vi "RPT_Report Calibrate.vi"(8 "template":path=path "C:/AllenProjects/PWC-OLS/$Calibrtation/CAL_Level_RnR_241105.xlsx", 9 "Info":cluster{"Name":string, "Date":string}[](array[cluster])=[{"Name"="Joe", "Date"="Today"}], 10 "LinEq":T1(array[cluster]), 11 "Calibration":cluster{"SP":dbl, "Laser":dbl, "Measure":dbl}[](array[cluster])=[{"SP"=2.0, "Laser"=2.0014999999999996, "Measure"=2.0}, {"SP"=3.5, "Laser"=3.5015, "Measure"=3.5}, {"SP"=5.0, "Laser"=5.001499999999945, "Measure"=5.0}, {"SP"=6.5, "Laser"=6.50149999999989, "Measure"=6.5}, {"SP"=8.0, "Laser"=8.001499999999835, "Measure"=8.0}]) -> ()   [LabVIEW 2024]
uses:
  <vilib>/Utility/NIReport.llb/Report Type.ctl
  <vilib>/addons/_office/excel.llb/Excel Easy Table (str).vi
  <vilib>/Utility/NIReport.llb/NI_report.lvclass
  <vilib>/Utility/NIReport.llb/NI_ReportGenerationCore.lvlib
  <vilib>/Utility/NIReport.llb/Excel/NI_Excel.lvclass
  <vilib>/addons/_office/NI_ReportGenerationToolkit.lvlib
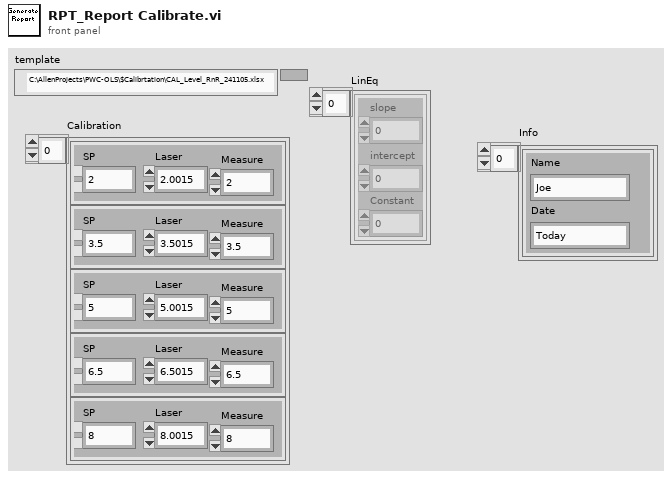
[diagram p1: front panel]
types:
  T1 = cluster{"slope":dbl, "intercept":dbl, "Constant":dbl}[]
  T2 = typedef "NI_ReportGenerationCore.lvlib/Report Type.ctl" = enum16{"HTML", "Word", "Excel"}
  T3 = cluster{"position (excel)":cluster{"row":i32, "column":i32}, "name (excel)":string, "bookmark (word)":string}
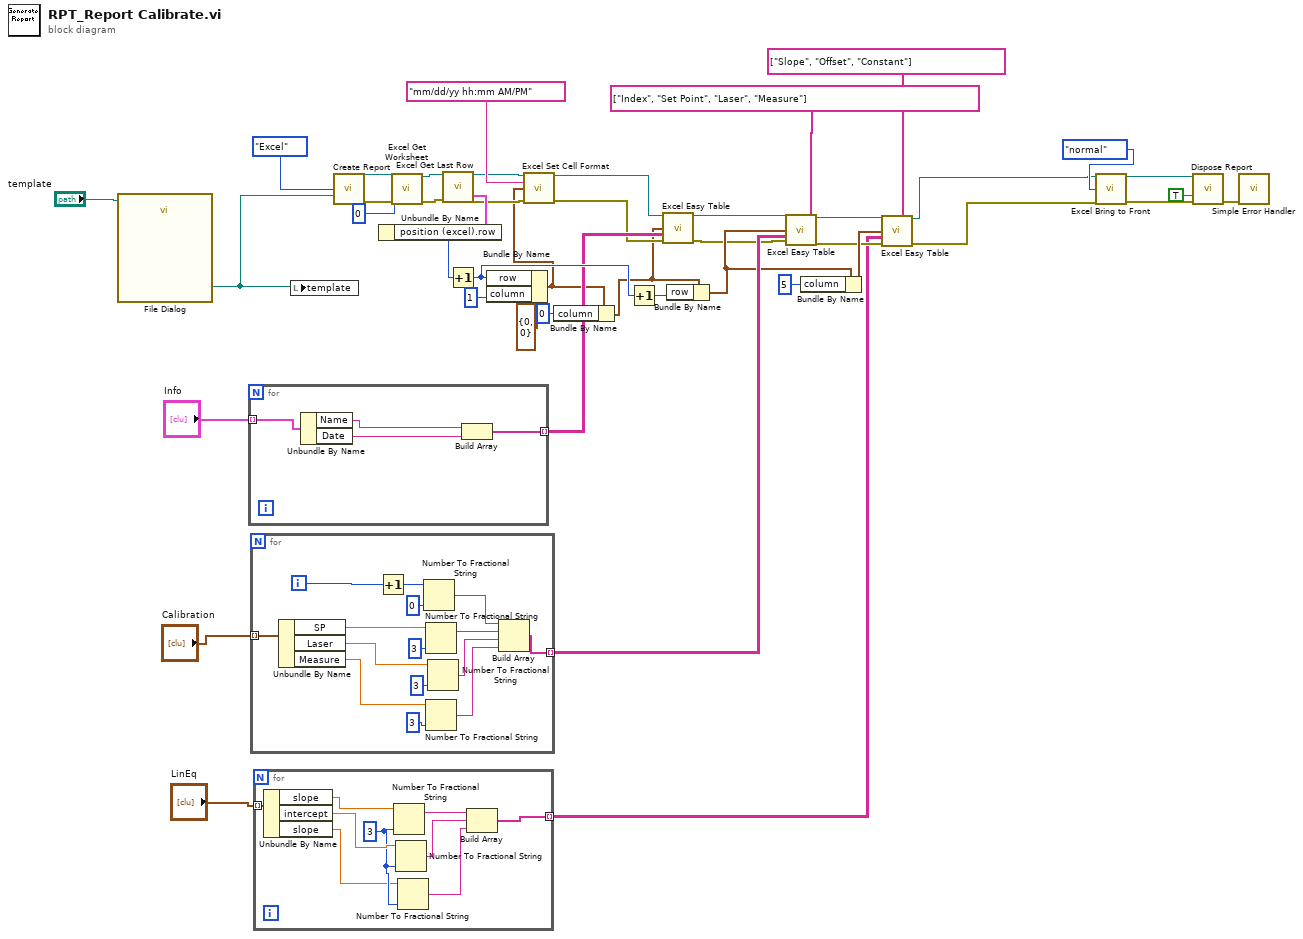
[diagram p0: block diagram]
diagram:
  n1 = call "File Dialog"("start path"="template") -> ("selected path"=w19:path)  [unwired: 11 in, 3 out]
  n2 = for {
    tunnel: [w48] -> w10 mode=indexing
    tunnel: "Info" -> [w47] mode=indexing
    n3 = Unbundle By Name(w47) -> ("Name"=w46:string, "Date"=w45:string)
    n4 = Build Array(w46, w45) -> (w48:string[])
  }
  n5 = for {
    tunnel: "Calibration" -> [w54] mode=indexing
    tunnel: [w49] -> w27 mode=indexing
    i -> [w53]
    n6 = Unbundle By Name(w54) -> ("SP"=w52:dbl, "Laser"=w51:dbl, "Measure"=w50:dbl)
    n7 = Increment(x=w53) -> (x+1=w56:i32)
    n8 = Number To Fractional String(number=w56, precision (6)=i16 0) -> (F-format string=w55:string)  [unwired: 2 in]
    n9 = Number To Fractional String(number=w52, precision (6)=i16 3) -> (F-format string=w60:string)  [unwired: 2 in]
    n10 = Number To Fractional String(number=w50, precision (6)=i16 3) -> (F-format string=w58:string)  [unwired: 2 in]
    n11 = Number To Fractional String(number=w51, precision (6)=i16 3) -> (F-format string=w59:string)  [unwired: 2 in]
    n12 = Build Array(w55, w60, w59, w58) -> (w49:string[])
  }
  n13 = for {
    tunnel: [w68] -> w22 mode=indexing
    tunnel: "LinEq" -> [w67] mode=indexing
    w65 = i16 3 ("precision (6)")
    n14 = Unbundle By Name(w67) -> ("slope"=w70:dbl, "intercept"=w69:dbl, "slope"=w64:dbl)
    n15 = Number To Fractional String(number=w70, precision (6)=w65) -> (F-format string=w72:string)  [unwired: 2 in]
    n16 = Number To Fractional String(number=w69, precision (6)=w65) -> (F-format string=w71:string)  [unwired: 2 in]
    n17 = Number To Fractional String(number=w64, precision (6)=w65) -> (F-format string=w66:string)  [unwired: 2 in]
    n18 = Build Array(w72, w71, w66) -> (w68:string[])
  }
  n19 = local write "template"(w19) -> ()
  n20 = call <vilib>:"Create Report.vi"("report type"=Report_Type."Excel" ("Report Type"), "template (empty)"=w19) -> ("report out"=w34:refnum<class "NI_report.lvclass">, "error out"=w33:errorcluster)  [unwired: 12 in]
  n21 = call <vilib>:"Excel Get Worksheet.vi"("report in"=w34, "worksheet index (0)"=0, "error in (no error)"=w33) -> ("report out"=w37:refnum<class "NI_report.lvclass">, "error out"=w36:errorcluster)  [unwired: 11 in]
  n22 = call <vilib>:"Excel Get Last Row.vi"("report in"=w37, "error in (no error)"=w36) -> ("report out"=w8:refnum<class "NI_report.lvclass">, "MS Office parameters out"=w32:T3, "error out"=w7:errorcluster)  [unwired: 11 in]
  n23 = Unbundle By Name(w32) -> ("position (excel).row"=w31:i32)
  n24 = Increment(x=w31) -> (x+1=w13:i32)
  n25 = Bundle By Name(cluster=cluster{"row":i32, "column":i32} {"row"=0, "column"=0} ("start (0, 0)"), "row"=w13, "column"=1) -> (w2:cluster{"row":i32, "column":i32})
  n26 = call <vilib>:"Excel Set Cell Format.vi"("report in"=w8, "number format"="mm/dd/yy hh:mm AM/PM", "start (-1, -1)"=w2, "error in (no error)"=w7) -> ("report out"=w6:refnum<class "NI_report.lvclass">, "error out"=w5:errorcluster)  [unwired: 10 in]
  n27 = Bundle By Name(cluster=w2, "column"=0) -> (w4:cluster{"row":i32, "column":i32})
  n28 = Increment(x=w13) -> (x+1=w14:i32)
  n29 = call-poly <vilib>:"Excel Easy Table.vi"("report in"=w6, "start (0, 0)"=w4, "text data"=w10, "error in (no error)"=w5) -> ("report out"=w12:refnum<class "NI_report.lvclass">, "error out"=w11:errorcluster)  [unwired: 7 in, 3 out]
  n30 = Bundle By Name(cluster=w4, "row"=w14) -> (w15:cluster{"row":i32, "column":i32})
  n31 = call-poly <vilib>:"Excel Easy Table.vi"("report in"=w12, "start (0, 0)"=w15, "text data"=w27, "error in (no error)"=w11, "column headers"=string[] ["Index", "Set Point", "Laser", "Measure"] ("row headers")) -> ("report out"=w25:refnum<class "NI_report.lvclass">, "error out"=w24:errorcluster)  [unwired: 6 in, 3 out]
  n32 = Bundle By Name(cluster=w15, "column"=5) -> (w26:cluster{"row":i32, "column":i32})
  n33 = call-poly <vilib>:"Excel Easy Table.vi"("report in"=w25, "start (0, 0)"=w26, "text data"=w22, "error in (no error)"=w24, "column headers"=string[] ["Slope", "Offset", "Constant"] ("Array 2")) -> ("report out"=w21:refnum<class "NI_report.lvclass">, "error out"=w20:errorcluster)  [unwired: 6 in, 3 out]
  n34 = call <vilib>:"Excel Bring to Front.vi"("report in"=w21, "window state (maximized)"=enum16{"maximized", "minimized", "normal"}."normal", "error in (no error)"=w20) -> ("report out"=w41:refnum<class "NI_report.lvclass">, "error out"=w42:errorcluster)  [unwired: 11 in]
  n35 = call-dynamic "Dispose Report.vi"("report in"=w41, "save changes? (F)"=TRUE, "error in (no error)"=w42) -> ("error out"=w40:errorcluster)  [unwired: 12 in]
  n36 = call <vilib>:"Simple Error Handler.vi"("error in (no error)"=w40) -> ()  [unwired: 4 in, 5 out]
